vi "SimpleBatteryState_Sub.vi"() -> (3 "Enum":T1)   [LabVIEW 2021]
uses:
  States_Enum.ctl
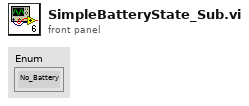
[diagram p1: front panel]
types:
  T1 = typedef "States_Enum.ctl" = enum16{"No_Battery", "Battery_Inserted", ""}
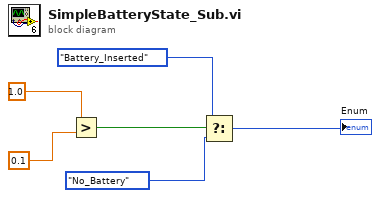
[diagram p0: block diagram]
diagram:
  n1 = Greater?(x=1.0, y=0.1) -> (0:w3:bool)
  n2 = Select(t=States_Enum."Battery_Inserted", s=w3, f=States_Enum."No_Battery") -> (s? t:f=→"Enum":T1)
